vi "PH_AxisGUI_NF.ProcCases.vi"(0 "i ref in":refnum<vi>, 1 "selector":string, 2 "data":i8[](array[numeric]), 3 "call cluster":T1={"Object"="", "Selector"="", "CallType"=enum."synchronous", "Async Object"="", "Async Selector"="", "Data Descriptor"="", "Data"=[], "Error #"=0, "Expire"=0}, 5 "error in":errorcluster) -> (14 "i ref out":refnum<vi>, 17 "answer cluster":T1={"Object"="", "Selector"="", "CallType"=enum."synchronous", "Async Object"="", "Async Selector"="", "Data Descriptor"="", "Data"=[], "Error #"=0, "Expire"=0}, 19 "error out":errorcluster)   [LabVIEW 2014, in "PH_AxisGUI_NF.lvlib"]
doc: "This method is called by a process from within the default case in the event loop. The methods of a class that are linked to events will be called from THIS method. Add your code here."
uses:
  PH_AxisGUI_NF.lvlib
  CS_Core/CSSystem/CoreDefs/CoreDefs.call_type.ctl
  CS_Core/BaseProcess/BaseProcess.descriptor string definition.ctl
  CS_Core/CSSystem/CoreDefs/CoreDefs.rawDataType.ctl
  CS_Core/CSSystem/CoreLib/CoreLib.string 2 byte array.vi
  CS_Core/BaseProcess/BaseProcess.lvlib
  CS_Core/CSSystem/CoreLib/CoreLib.lvlib
  PH_Basics/PH_StatusHandler/PH_StatusHandler.lvlib
  CS_Core/CAEObj/CAEObj.lvlib
  PH_Basics/PH_Common/PH_Common.lvlib
  PH_Basics/PH_Class/PH_Class.lvlib
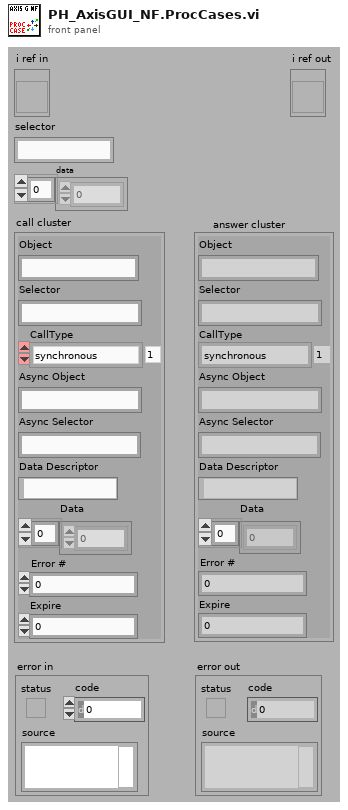
[diagram p1: front panel]
types:
  T1 = typedef "CoreDefs.call_type.ctl" = cluster{"Object":string, "Selector":string, "CallType":enum16{"simple", "synchronous", "asynchronous"}, "Async Object":string, "Async Selector":string, "Data Descriptor":T2, "Data":T3, "Error #":i32, "Expire":u32}
  T2 = typedef "BaseProcess.lvlib/BaseProcess.descriptor string definition.ctl" = string
  T3 = typedef "CoreDefs.rawDataType.ctl" = i8[]
  T4 = typedef "PH_StatusHandler.lvlib/PH_StatusHandler.Status.ctl" = i16
  T5 = typedef "PH_AxisGUI_NF.lvlib/PH_AxisGUI_NF.i attribute.ctl" = cluster{"GUI Refs":cluster{"Delete":refnum<vi>, "Slide 0":refnum<vi>, "Slide 1":refnum<vi>, "Slide 2":refnum<vi>, "Instance Status":refnum<vi>, "Position":refnum<vi>, "Reset":refnum<vi>, "Goal":refnum<vi>, "Go":refnum<vi>}, "Instance":string, "Name Axis 0":string, "Name Axis 1":string, "Name Axis 2":string, "System":string, "Driver Type":T6, "Offset":i32, "Goal":i32}
  T6 = typedef "NF87XX.lvlib/NF87XX.driver Type.ctl" = enum16{"not defined", "3-ch open loop drv", "1-ch closed loop drv"}
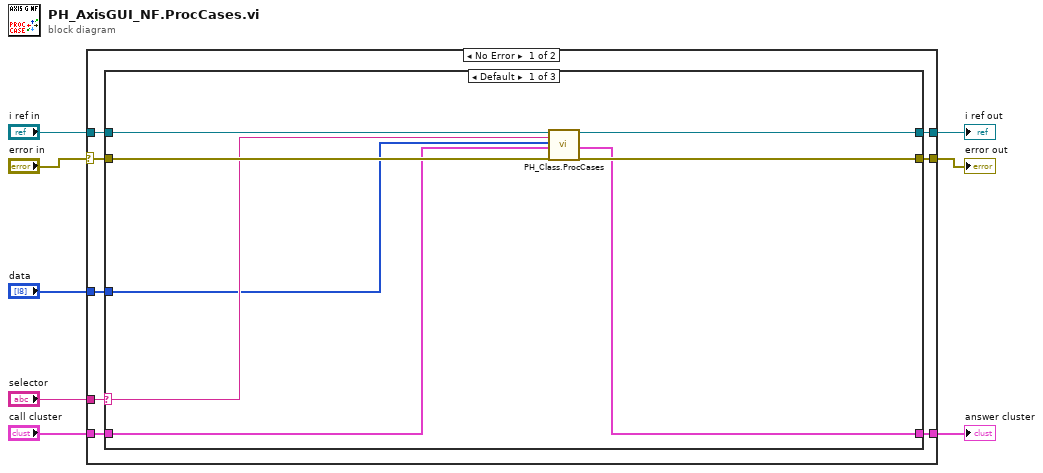
[diagram p0: block diagram]
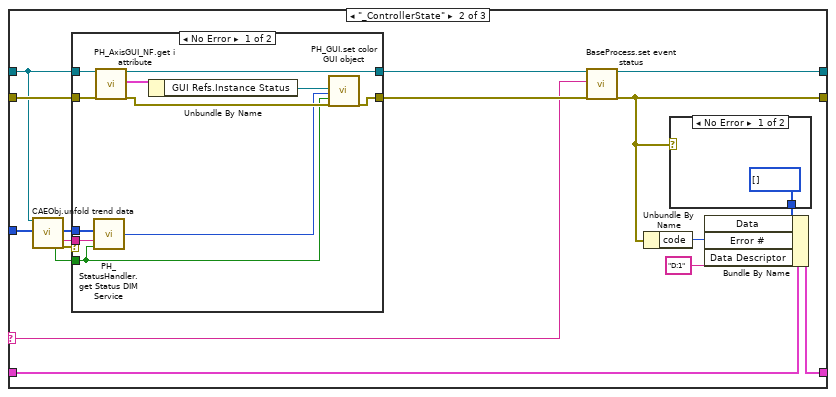
[diagram p2: hidden frame]
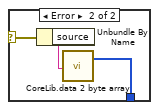
[diagram p3: hidden frame]
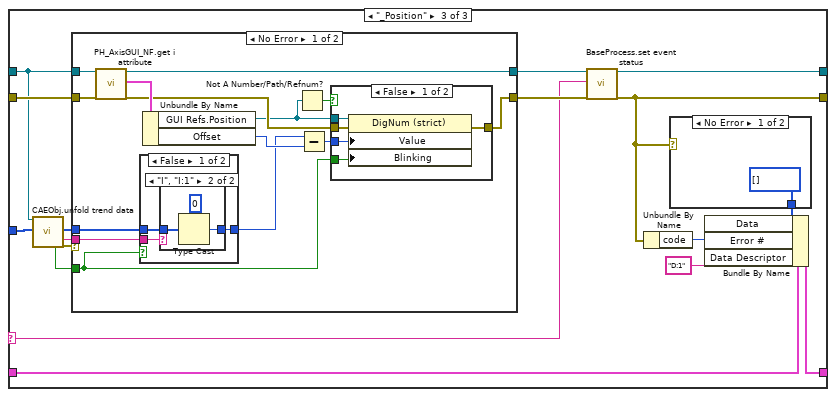
[diagram p5: hidden frame]
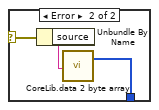
[diagram p6: hidden frame]
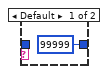
[diagram p7: hidden frame]
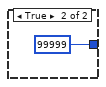
[diagram p8: hidden frame]
diagram:
  n1 = case shown="No Error" "error in" {
    selector: "error in" -> [w10 w111]
    tunnel: "selector" -> [w16 _]
    tunnel: [w15 w110] -> w7
    tunnel: "call cluster" -> [w14 w110]
    tunnel: "i ref in" -> [w13 w112]
    tunnel: [w12 w112] -> w4
    tunnel: [w9 w111] -> w3
    tunnel: "data" -> [w11 _]
    frame No Error {
      n2 = case shown="Default" w16 {
        selector: w16 -> [w19 w38 w72]
        tunnel: w13 -> [w18 w31 w65]
        tunnel: [w24 w37 w71] -> w12
        tunnel: w14 -> [w20 w26 w60]
        tunnel: [w21 w25 w59] -> w15
        tunnel: w10 -> [w23 w41 w75]
        tunnel: w11 -> [w17 w32 w66]
        tunnel: [w22 w33 w67] -> w9
        frame Default {
          n3 = call "PH_Class.ProcCases.vi"("i ref in"=w18, "selector"=w19, "Data"=w17, "call cluster"=w20, "error in (no error)"=w23) -> ("i ref out"=w24:refnum<vi>, "answer cluster"=w21:T1, "error out"=w22:errorcluster)  [unwired: 12 in]
        }
        frame "_ControllerState" {
          n4 = call "CAEObj.unfold trend data.vi"("i ref in"=w31, "raw trend data"=w32) -> ("no link"=w27:bool, "data"=w29:i8[], "typeDescriptor"=w28:string, "error out"=w30:errorcluster)  [unwired: 9 in, 5 out]
          n5 = case shown="No Error" w30 {
            tunnel: [w53 w58] -> w40
            tunnel: w31 -> [w54 w58]
            tunnel: w41 -> [w52 w57]
            tunnel: [w48 w57] -> w39
            tunnel: w29 -> [w56 _]
            tunnel: w28 -> [w55 _]
            tunnel: w27 -> [w47 _]
            frame No Error {
              n6 = call "PH_StatusHandler.get Status DIM Service.vi"("no link"=w47, "typeDescriptor"=w55, "data"=w56) -> ("Status"=w46:T4)  [unwired: 1 in]
              n7 = call "PH_AxisGUI_NF.get i attribute.vi"("i ref in"=w54, "error in (no error)"=w52) -> ("i ref out"=w53:refnum<vi>, "i attribute"=w51:T5, "error out"=w49:errorcluster)  [unwired: 15 in]
              n8 = Unbundle By Name(w51) -> ("GUI Refs.Instance Status"=w50:refnum<vi>)
              n9 = call "PH_GUI.set color GUI object.vi"("GUI object Ref"=w50, "State"=w46, "Blinking? (false)"=w47, "error in (no error)"=w49) -> ("error out"=w48:errorcluster)  [unwired: 15 in]
            }
            frame Error {
            }
          }
          n10 = call "BaseProcess.set event status.vi"("i ref in"=w40, "EventStatus"=w38, "error in (no error)"=w39) -> ("i ref out"=w37:refnum<vi>, "error out"=w33:errorcluster)  [unwired: 14 in, 1 out]
          n11 = Unbundle By Name(w33) -> ("code"=w36:i32)
          n12 = case shown="No Error" w33 {
            selector: w33 -> [_ w45]
            tunnel: [T3 [] ("byteArray out") w43] -> w34
            frame No Error {
            }
            frame Error {
              n13 = Unbundle By Name(w45) -> ("source"=w44:string)
              n14 = call-poly "CoreLib.data 2 byte array.vi"("string"=w44) -> ("byteArray out"=w43:T3)  [unwired: 18 in]
            }
          }
          n15 = Bundle By Name(cluster=w26, "Data"=w34, "Error #"=w36, "Data Descriptor"="D:1") -> (w25:T1)
        }
        frame "_Position" {
          n16 = call "CAEObj.unfold trend data.vi"("i ref in"=w65, "raw trend data"=w66) -> ("no link"=w61:bool, "data"=w63:i8[], "typeDescriptor"=w62:string, "error out"=w64:errorcluster)  [unwired: 9 in, 5 out]
          n17 = case shown="No Error" w64 {
            tunnel: [w92 w109] -> w74
            tunnel: w65 -> [w93 w109]
            tunnel: w75 -> [w91 w108]
            tunnel: [w88 w108] -> w73
            tunnel: w63 -> [w83 _]
            tunnel: w62 -> [w84 _]
            tunnel: w61 -> [w85 _]
            frame No Error {
              n18 = call "PH_AxisGUI_NF.get i attribute.vi"("i ref in"=w93, "error in (no error)"=w91) -> ("i ref out"=w92:refnum<vi>, "i attribute"=w90:T5, "error out"=w89:errorcluster)  [unwired: 15 in]
              n19 = case "No link?" shown="False" w85 {
                tunnel: [w96 99999] -> w80
                tunnel: w83 -> [w95 _]
                tunnel: w84 -> [w94 _]
                frame False {
                  n20 = case "Check data type" shown="\"I\", \"I:1\"" w94 {
                    tunnel: [99999 w98] -> w96
                    tunnel: w95 -> [_ w99]
                    frame Default {
                    }
                    frame "I", "I:1" {
                      n21 = Type Cast(type=0, x=w99) -> (*(type *) &x=w98:i32)
                    }
                  }
                }
                frame True {
                }
              }
              n22 = Unbundle By Name(w90) -> ("GUI Refs.Position"=w86:refnum<vi>, "Offset"=w82:i32)
              n23 = Not A Number/Path/Refnum?(number/path/refnum=w86) -> (NaN/Path/Refnum?=w87:bool)
              n24 = Subtract(x=w80, y=w82) -> (x-y=w81:i32)
              n25 = case shown="False" w87 {
                tunnel: w89 -> [w106 w107]
                tunnel: [w105 w107] -> w88
                tunnel: w86 -> [w104 _]
                tunnel: w85 -> [w103 _]
                tunnel: w81 -> [w102 _]
                frame False {
                  n26 = property class="DigNum (strict)"(reference=w104, error in=w106, "Value"=w102, "Blinking"=w103) -> (error out=w105:errorcluster)  [unwired: 1 out]
                }
                frame True {
                }
              }
            }
            frame Error {
            }
          }
          n27 = call "BaseProcess.set event status.vi"("i ref in"=w74, "EventStatus"=w72, "error in (no error)"=w73) -> ("i ref out"=w71:refnum<vi>, "error out"=w67:errorcluster)  [unwired: 14 in, 1 out]
          n28 = Unbundle By Name(w67) -> ("code"=w70:i32)
          n29 = case shown="No Error" w67 {
            selector: w67 -> [_ w79]
            tunnel: [T3 [] ("byteArray out") w77] -> w68
            frame No Error {
            }
            frame Error {
              n30 = Unbundle By Name(w79) -> ("source"=w78:string)
              n31 = call-poly "CoreLib.data 2 byte array.vi"("string"=w78) -> ("byteArray out"=w77:T3)  [unwired: 18 in]
            }
          }
          n32 = Bundle By Name(cluster=w60, "Data"=w68, "Error #"=w70, "Data Descriptor"="D:1") -> (w59:T1)
        }
      }
    }
    frame Error {
    }
  }
  "answer cluster" <- w7
  "i ref out" <- w4
  "error out" <- w3
